vi "Tower light.vi"(10 "Enum":enum16{"Green", "Red", "Yellow", "OFF"}(ring)) -> ()   [LabVIEW 2015]
uses:
  Galobal variable_TI.vi
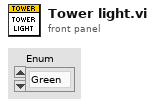
[diagram p1: front panel]
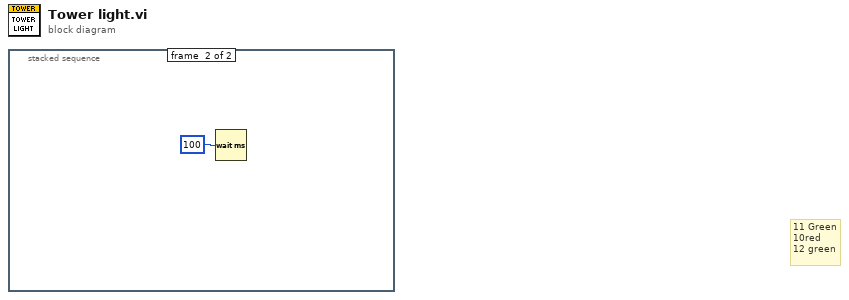
[diagram p0: block diagram]
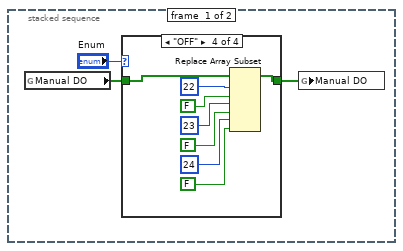
[diagram p2: hidden frame]
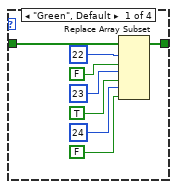
[diagram p3: hidden frame]
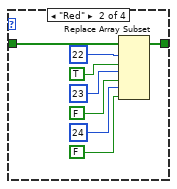
[diagram p4: hidden frame]
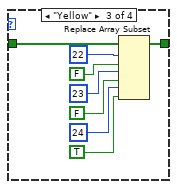
[diagram p5: hidden frame]
diagram:
  # "11 Green\n10red\n12 green"
  n1 = stacked-sequence {
    frame #0 {
      n2 = global read "Galobal variable_TI.vi" "Manual DO"() -> (w1:bool[])
      n3 = case shown="\"OFF\"" "Enum" {
        tunnel: w1 -> [w5 w15 w21 w30]
        tunnel: [w4 w12 w20 w29] -> w2
        frame "Green", Default {
          n4 = Replace Array Subset(array=w5, new element #1=FALSE ("new element/subarray"), index #1=22 ("index"), new element #2=TRUE ("new element/subarray"), index #2=23 ("index"), new element #3=FALSE ("new element/subarray"), index #3=24 ("index")) -> (w4:bool[])
        }
        frame "Red" {
          n5 = Replace Array Subset(array=w15, new element #1=TRUE ("new element/subarray"), index #1=22 ("index"), new element #2=FALSE ("new element/subarray"), index #2=23 ("index"), new element #3=FALSE ("new element/subarray"), index #3=24 ("index")) -> (w12:bool[])
        }
        frame "Yellow" {
          n6 = Replace Array Subset(array=w21, new element #1=FALSE ("new element/subarray"), index #1=22 ("index"), new element #2=FALSE ("new element/subarray"), index #2=23 ("index"), new element #3=TRUE ("new element/subarray"), index #3=24 ("index")) -> (w20:bool[])
        }
        frame "OFF" {
          n7 = Replace Array Subset(array=w30, new element #1=FALSE ("new element/subarray"), index #1=22 ("index"), new element #2=FALSE ("new element/subarray"), index #2=23 ("index"), new element #3=FALSE ("new element/subarray"), index #3=24 ("index")) -> (w29:bool[])
        }
      }
      n8 = global write "Galobal variable_TI.vi" "Manual DO"(w2) -> ()
    }
    frame #1 {
      n9 = Wait (ms)(milliseconds to wait=u32 100) -> ()  [unwired: 1 out]
    }
  }
